vi "Table Select Section Copy.vi"(11 "Table Ref In":refnum<vi>) -> (1 "Copied Value":string[][](array[string]), 3 "Table Ref Out":refnum<vi>)   [LabVIEW 2024]
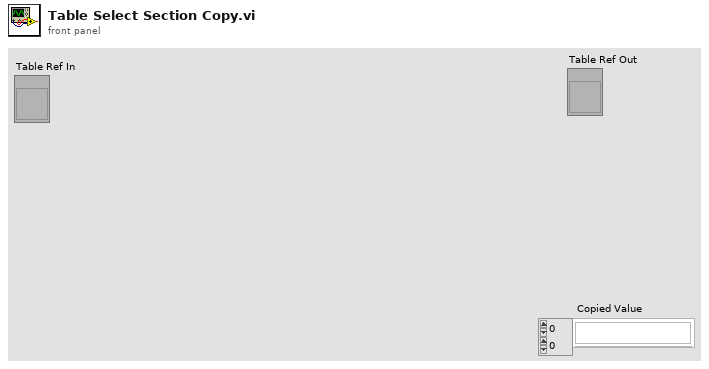
[diagram p1: front panel]
types:
  T1 = typedef "LVRowAndColumnTypeDef.ctl" = cluster{"Row":i32, "Column":i32}
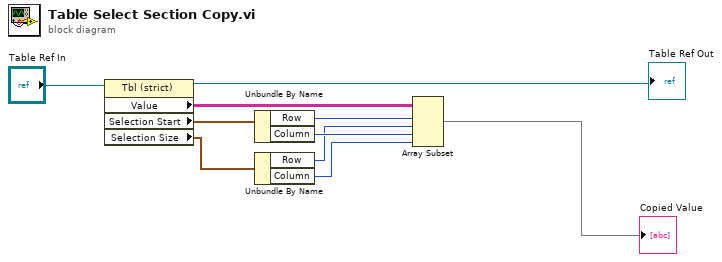
[diagram p0: block diagram]
diagram:
  n1 = property class="Tbl (strict)"(reference="Table Ref In") -> (reference out=→"Table Ref Out":refnum<vi>, "Value"=w7:string[][], "Selection Start"=w8:T1, "Selection Size"=w4:T1)  [unwired: 1 in, 1 out]
  n2 = Unbundle By Name(w8) -> ("Row"=w6:i32, "Column"=w5:i32)
  n3 = Unbundle By Name(w4) -> ("Row"=w3:i32, "Column"=w2:i32)
  n4 = Array Subset(array=w7, index (row)=w6, length (row)=w3, index (col)=w5, length (col)=w2) -> (→"Copied Value":string[][])
